vi "ArcadeDrive.vi"(8 "error in":errorcluster, 10 "Turn":dbl, 11 "Forward":dbl) -> (0 "error out":errorcluster)   [LabVIEW 2016]
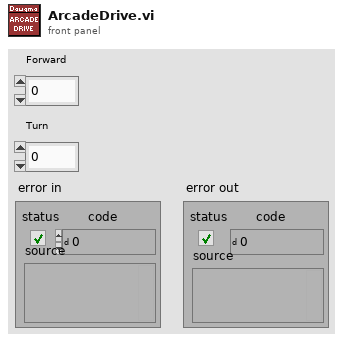
[diagram p1: front panel]
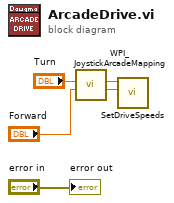
[diagram p0: block diagram]
diagram:
  n1 = call <vilib>:"WPI_JoystickArcadeMapping.vi"("Y axis value"="Forward", "X axis value"="Turn") -> ("Right Motor Value"=w2:dbl, "Left Motor Value"=w1:dbl)  [unwired: 8 in]
  n2 = call "SetDriveSpeeds.vi"("Right Value"=w2, "Left Value"=w1) -> ()  [unwired: 9 in, 1 out]
  "error out" <- "error in"
